vi "Thorlabs-Acquire Next Image.vi"(8 "error in (no error)":errorcluster, 11 "pDataBuffer in":u16[](array[numeric])) -> (0 "error out":errorcluster, 3 "pDataBuffer out":u16[](array[numeric]), 4 "Aq Iter":i32)   [LabVIEW 2020]
uses:
  LSM_SDK/ThorConfocal.lvlib
  ECU_SDK/ThorECU.lvlib
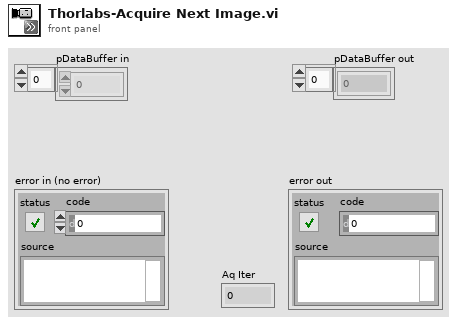
[diagram p1: front panel]
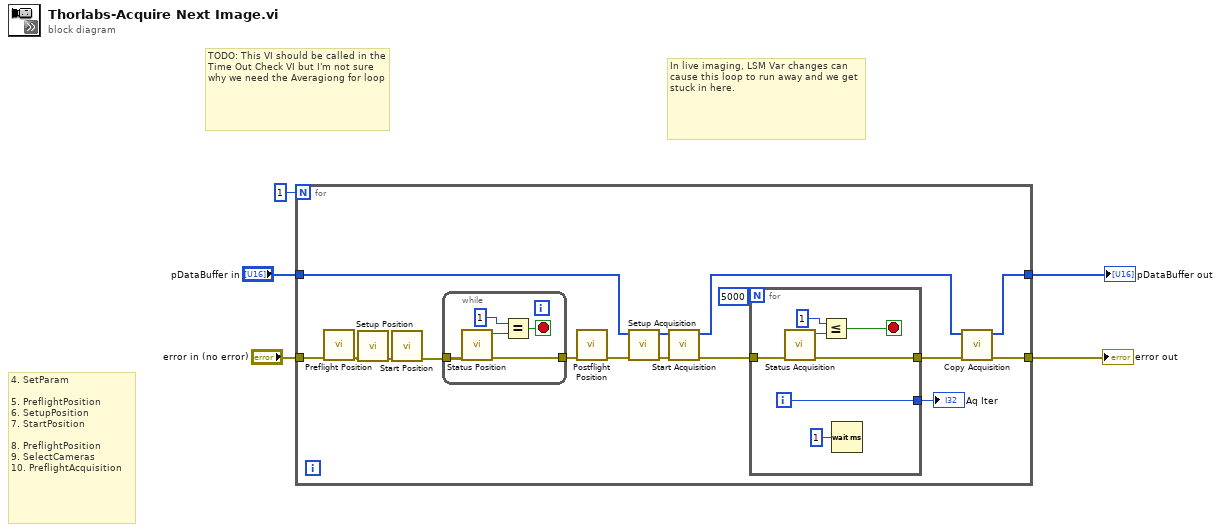
[diagram p0: block diagram]
diagram:
  # "TODO: This VI should be called in the Time Out Check VI but I'm not sure why we need the Averagiong for loop"
  # "4. SetParam\n\n5. PreflightPosition\n6. SetupPosition\n7. StartPosition\n\n8. PreflightPosition\n9. SelectCameras\n10. PreflightAcquisition"
  # "In live imaging, LSM Var changes can cause this loop to run away and we get stuck in here."
  n1 = for {
    N: 1 -> [_]
    tunnel: "pDataBuffer in" -> [w8]
    tunnel: [w20] -> w4
    tunnel: "error in (no error)" -> [w10]
    tunnel: [w21] -> w5
    n2 = call "Preflight Position.vi"("error in (no error)"=w10) -> ("error out"=w15:errorcluster)  [unwired: 9 in, 1 out]
    n3 = call "Setup Position.vi"("error in (no error)"=w15) -> ("error out"=w16:errorcluster)  [unwired: 9 in, 1 out]
    n4 = call "Start Position.vi"("error in (no error)"=w16) -> ("error out"=w14:errorcluster)  [unwired: 9 in, 1 out]
    n5 = while {
      tunnel: w14 -> [w33]
      tunnel: [w32] -> w13
      stop <- w30 stop-if-true
      n6 = call "Status Position.vi"("error in (no error)"=w33) -> ("error out"=w32:errorcluster, "status out"=w29:i32)  [unwired: 8 in, 1 out]
      n7 = Equal?(x=1, y=w29) -> (x = y?=w30:bool)
    }
    n8 = call "Postflight Position.vi"("error in (no error)"=w13) -> ("error out"=w12:errorcluster)  [unwired: 9 in, 1 out]
    n9 = call "Setup Acquisition.vi"("error in (no error)"=w12, "pDataBuffer"=w8) -> ("error out"=w18:errorcluster, "pDataBuffer"=w11:u16[])  [unwired: 3 in, 1 out]
    n10 = call "Start Acquisition.vi"("error in (no error)"=w18, "pDataBuffer"=w11) -> ("error out"=w17:errorcluster, "pDataBuffer"=w7:u16[])  [unwired: 3 in, 1 out]
    n11 = for {
      N: 5000 ("Timeout for StatusAcquisition") -> [_]
      tunnel: [w25] -> w19
      tunnel: w17 -> [w28]
      tunnel: [w24] -> w9
      i -> [w24]
      stop <- w23 stop-if-true
      n12 = call "Status Acquisition.vi"("error in (no error)"=w28) -> ("error out"=w25:errorcluster, "status out"=w26:i32)  [unwired: 4 in, 1 out]
      n13 = Less Or Equal?(x=1, y=w26) -> (x <= y?=w23:bool)
      n14 = Wait (ms)(milliseconds to wait=u32 1) -> ()  [unwired: 1 out]
    }
    "Aq Iter" <- w9
    n15 = call "Copy Acquisition.vi"("error in (no error)"=w19, "pDataBuffer"=w7) -> ("error out"=w21:errorcluster, "pDataBuffer"=w20:u16[])  [unwired: 3 in, 1 out]
  }
  "error out" <- w5
  "pDataBuffer out" <- w4
